vi "nii_read_data.vi"(8 "error in (no error)":errorcluster, 11 "file (use dialog)":path) -> (0 "error out":errorcluster, 2 "data value reference":refnum<data-value>, 3 "Data":T1 {"slice orientation" items=["transverse unflipped", "coronal unflipped", "sagittal unflipped", "transverse flipped", "coronal flipped", "sagittal flipped"]}, 4 "non-flip":bool, 5 "head":u8[](array[numeric]) format="%.0x")   [LabVIEW 2014]
uses:
  control/head_data.ctl
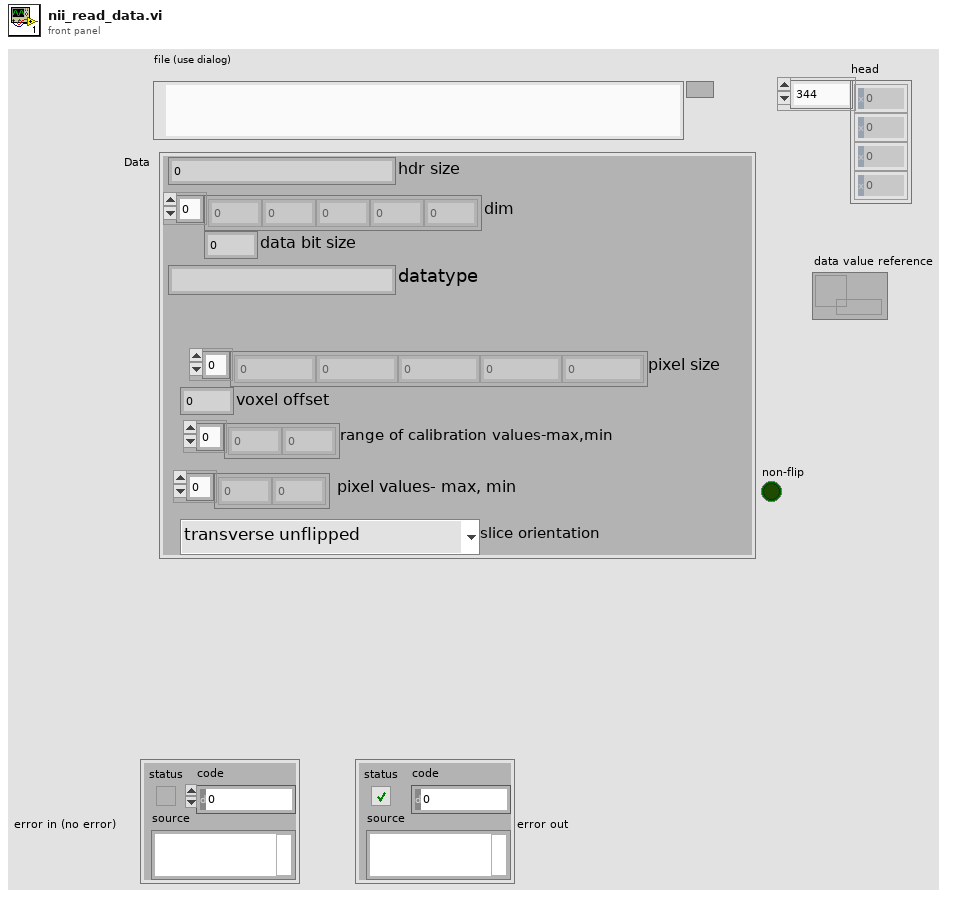
[diagram p1: front panel]
types:
  T1 = typedef "head_data.ctl" = cluster{"hdr size":i32, "dim":i32[], "data bit size":i32, "datatype":string, "pixel size ":sgl[], "voxel offset":sgl, "range of calibration values-max,min":sgl[], " pixel values- max, min":sgl[], "slice orientation":u16}
  T2 = enum16{"u_int8", "int8", "u_int16", "int16", "u_int32", "int32", "u_int64", "int64", "float", "double"}
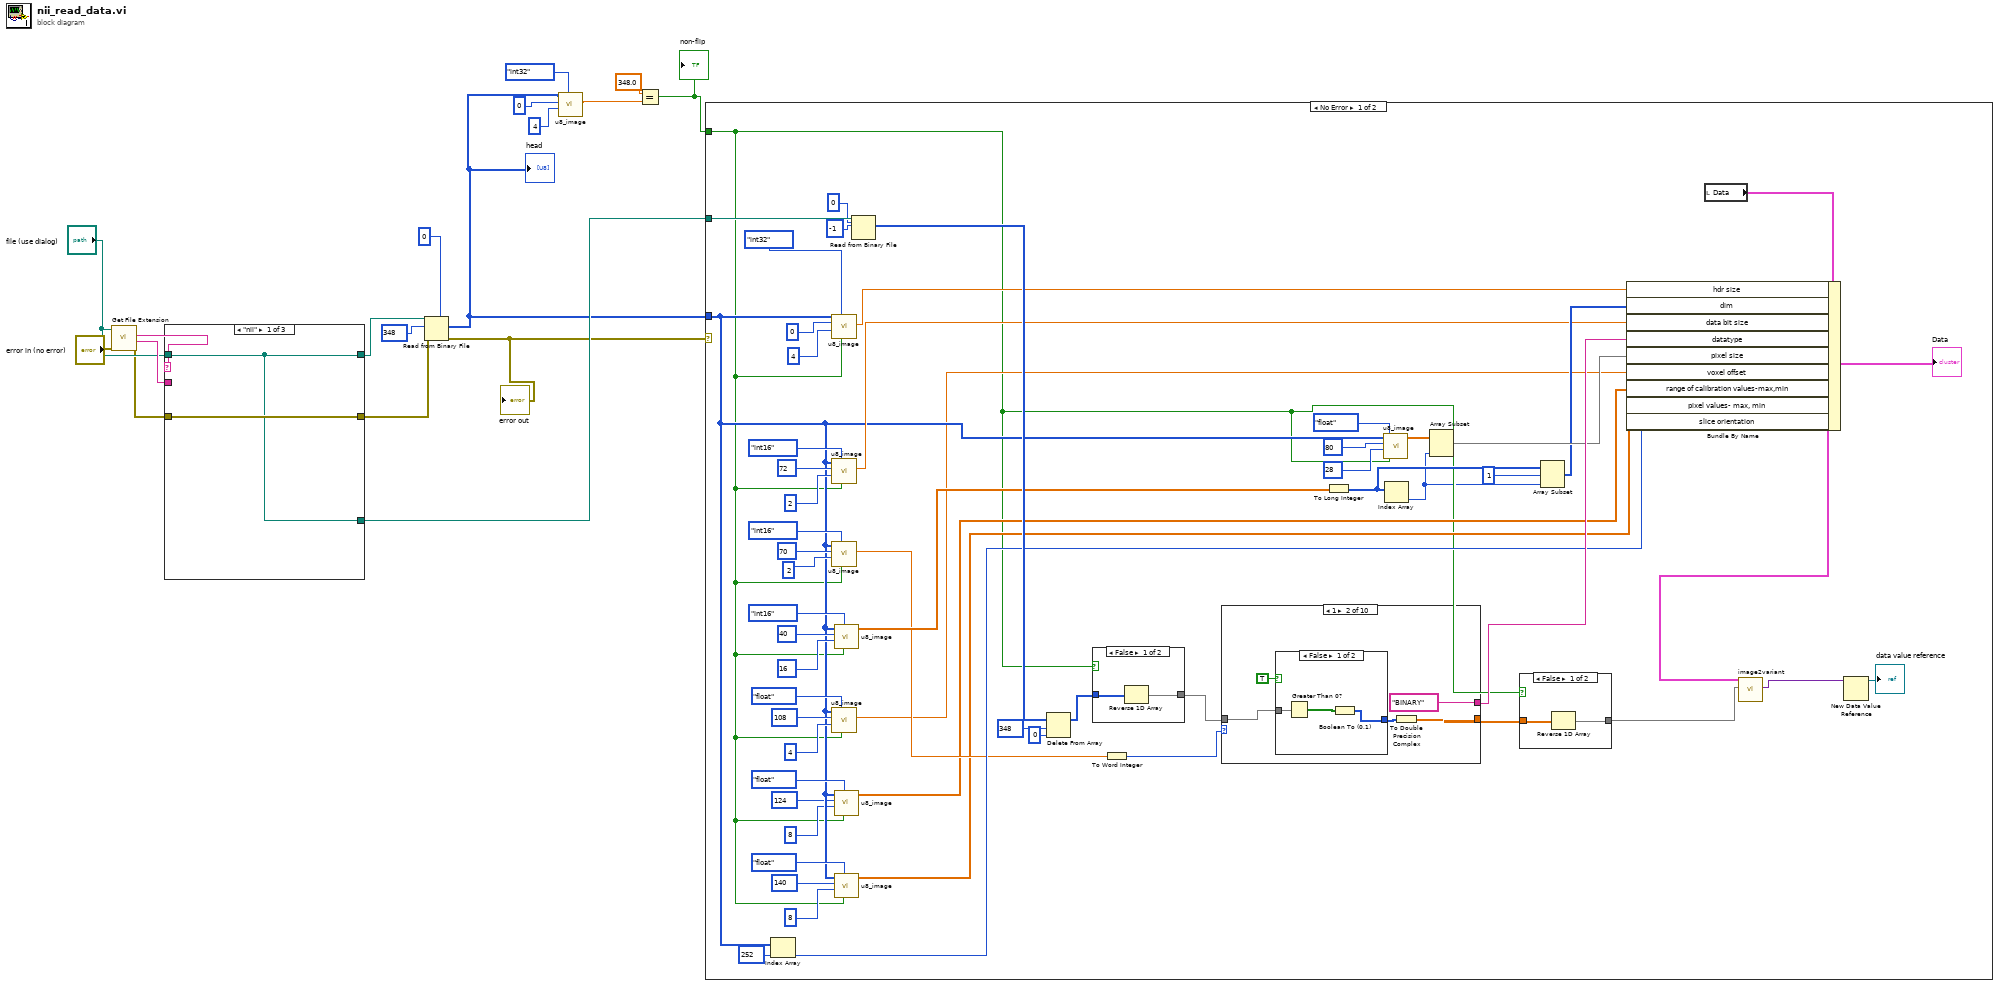
[diagram p0: block diagram]
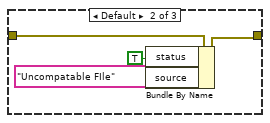
[diagram p2: hidden frame]
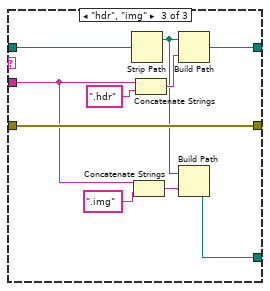
[diagram p3: hidden frame]
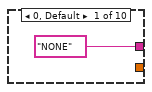
[diagram p6: hidden frame]
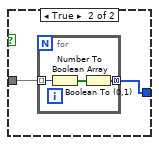
[diagram p7: hidden frame]
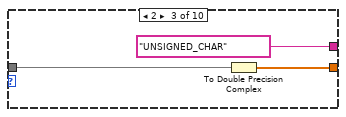
[diagram p8: hidden frame]
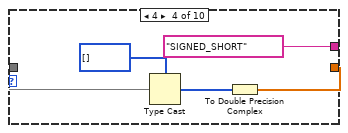
[diagram p9: hidden frame]
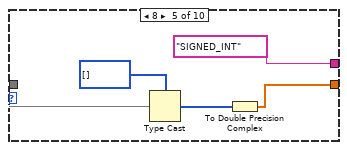
[diagram p10: hidden frame]
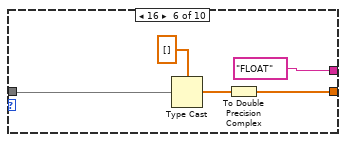
[diagram p11: hidden frame]
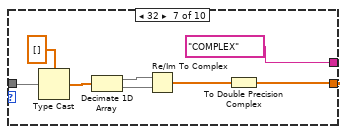
[diagram p12: hidden frame]
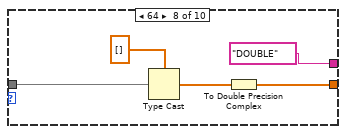
[diagram p13: hidden frame]
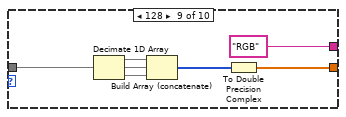
[diagram p14: hidden frame]
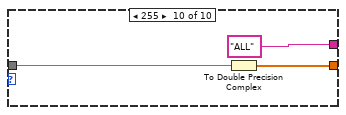
[diagram p15: hidden frame]
diagram:
  n1 = call <vilib>:"Get File Extension.vi"("error in (no error)"="error in (no error)", "file"="file (use dialog)") -> ("error out"=w14:errorcluster, "filename without extension"=w17:string, "lowercase file extension"=w18:string)  [unwired: 6 in, 1 out]
  n2 = case shown="\"nii\"" w18 {
    tunnel: "file (use dialog)" -> [w19 _ w30]
    tunnel: [w19 _ w32] -> w10
    tunnel: w17 -> [_ _ w26]
    tunnel: [w20 w23 w31] -> w15
    tunnel: w14 -> [w20 w24 w31]
    tunnel: [w19 _ w25] -> w12
    frame "nii" {
    }
    frame Default {
      n3 = Bundle By Name(cluster=w24, "status"=TRUE, "source"="Uncompatable FIle") -> (w23:errorcluster)
    }
    frame "hdr", "img" {
      n4 = Strip Path(path=w30) -> (stripped path=w29:path)  [unwired: 1 out]
      n5 = Concatenate Strings(w26, ".img" ("string")) -> (w28:string)
      n6 = Concatenate Strings(w26, ".hdr" ("string")) -> (w33:string)
      n7 = Build Path(base path=w29, name or relative path=w33) -> (appended path=w32:path)
      n8 = Build Path(base path=w29, name or relative path=w28) -> (appended path=w25:path)
    }
  }
  n9 = Read from Binary File(5:u8 0, 8:w15, 10:348 ("count (1)"), 11:w10) -> (0:w9:errorcluster, 2:w5:u8[])  [unwired: 2 in, 2 out]
  "error out" <- w9
  "head" <- w5
  n10 = call "u8_image.vi"("Enum"=T2."int32", "length"=4, "index"=0, "array"=w5) -> ("Numeric"=w3:dbl)  [unwired: 6 in, 1 out]
  n11 = Equal?(x=348.0, y=w3) -> (x = y?=w6:bool)
  "non-flip" <- w6
  n12 = case shown="No Error" w9 {
    tunnel: w5 -> [w49 _]
    tunnel: w12 -> [w91 _]
    tunnel: w6 -> [w41 _]
    frame No Error {
      n13 = Index Array(array=w49, index=252) -> (element=w83:u8)
      n14 = call "u8_image.vi"("non-flip"=w41, "Enum"=T2."int32", "length"=4, "index"=0, "array"=w49) -> ("Numeric"=w77:dbl)  [unwired: 5 in, 1 out]
      n15 = call "u8_image.vi"("non-flip"=w41, "Enum"=T2."int16", "length"=2, "index"=72, "array"=w49) -> ("Numeric"=w68:dbl)  [unwired: 5 in, 1 out]
      n16 = call "u8_image.vi"("non-flip"=w41, "Enum"=T2."int16", "length"=2, "index"=70, "array"=w49) -> ("Numeric"=w64:dbl)  [unwired: 5 in, 1 out]
      n17 = call "u8_image.vi"("non-flip"=w41, "Enum"=T2."float", "length"=4, "index"=108, "array"=w49) -> ("Numeric"=w46:dbl)  [unwired: 5 in, 1 out]
      n18 = call "u8_image.vi"("non-flip"=w41, "Enum"=T2."int16", "length"=16, "index"=40, "array"=w49) -> ("Array"=w74:dbl[])  [unwired: 5 in, 1 out]
      n19 = call "u8_image.vi"("non-flip"=w41, "Enum"=T2."float", "length"=8, "index"=124, "array"=w49) -> ("Array"=w50:dbl[])  [unwired: 5 in, 1 out]
      n20 = call "u8_image.vi"("non-flip"=w41, "Enum"=T2."float", "length"=8, "index"=140, "array"=w49) -> ("Array"=w53:dbl[])  [unwired: 5 in, 1 out]
      n21 = Read from Binary File(5:u8 0 ("default value 1"), 10:-1 ("count (1)"), 11:w91) -> (2:w88:u8[])  [unwired: 3 in, 3 out]
      n22 = Delete From Array(array=w88, length=348, index=0) -> (array with subset deleted=w44:u8[])  [unwired: 1 out]
      n23 = case shown="False" w41 {
        tunnel: [w95 w97] -> w43
        tunnel: w44 -> [w96 w97]
        frame False {
          n24 = Reverse 1D Array(array=w96) -> (reversed array=w95:u8[])
        }
        frame True {
        }
      }
      n25 = To Word Integer(number=w64) -> (16bit integer=w63:i16)
      n26 = case shown="1" w63 {
        tunnel: ["NONE" "BINARY" "UNSIGNED_CHAR" "SIGNED_SHORT" "SIGNED_INT" "FLOAT" "COMPLEX" "DOUBLE" "RGB" "ALL"] -> w87
        tunnel: [_ w102 w113 w118 w123 w128 w133 w141 w144 w150] -> w42
        tunnel: w43 -> [_ w101 w112 w117 w121 w125 w130 w138 w145 w151]
        frame 0, Default {
        }
        frame 1 {
          n27 = case shown="False" TRUE {
            tunnel: w101 -> [w105 w108]
            tunnel: [w104 w107] -> w100
            frame False {
              n28 = Greater Than 0?(x=w105) -> (x > 0?=w106:bool[])
              n29 = Boolean To (0,1)(Boolean=w106) -> (0, 1=w104:i16[])
            }
            frame True {
              n30 = for {
                tunnel: w108 -> [w111] mode=indexing
                tunnel: [w109] -> w107 mode=concatenating
                n31 = Number To Boolean Array(number=w111) -> (Boolean array=w110:bool[])
                n32 = Boolean To (0,1)(Boolean=w110) -> (0, 1=w109:i16[])
              }
            }
          }
          n33 = To Double Precision Complex(1:w100) -> (0:w102:cdb[])
        }
        frame 2 {
          n34 = To Double Precision Complex(1:w112) -> (0:w113:cdb[])
        }
        frame 4 {
          n35 = Type Cast(type=i16[] [], x=w117) -> (*(type *) &x=w116:i16[])
          n36 = To Double Precision Complex(1:w116) -> (0:w118:cdb[])
        }
        frame 8 {
          n37 = Type Cast(type=i32[] [], x=w121) -> (*(type *) &x=w120:i32[])
          n38 = To Double Precision Complex(1:w120) -> (0:w123:cdb[])
        }
        frame 16 {
          n39 = Type Cast(type=sgl[] [], x=w125) -> (*(type *) &x=w126:sgl[])
          n40 = To Double Precision Complex(1:w126) -> (0:w128:cdb[])
        }
        frame 32 {
          n41 = Type Cast(type=sgl[] [], x=w130) -> (*(type *) &x=w131:sgl[])
          n42 = Decimate 1D Array(w131) -> (w136:sgl[], w135:sgl[])
          n43 = Re/Im To Complex(1:w135, 2:w136) -> (0:w134:csg[])
          n44 = To Double Precision Complex(1:w134) -> (0:w133:cdb[])
        }
        frame 64 {
          n45 = Type Cast(type=dbl[] [], x=w138) -> (*(type *) &x=w139:dbl[])
          n46 = To Double Precision Complex(1:w139) -> (0:w141:cdb[])
        }
        frame 128 {
          n47 = Decimate 1D Array(w145) -> (w148:u8[], w147:u8[], w146:u8[])
          n48 = Build Array (concatenate)(w148, w147, w146) -> (w143:u8[])
          n49 = To Double Precision Complex(1:w143) -> (0:w144:cdb[])
        }
        frame 255 {
          n50 = To Double Precision Complex(1:w151) -> (0:w150:cdb[])
        }
      }
      n51 = To Long Integer(number=w74) -> (32bit integer=w80:i32[])
      n52 = call "u8_image.vi"("non-flip"=w41, "Enum"=T2."float", "length"=28, "index"=80, "array"=w49) -> ("Array"=w60:dbl[])  [unwired: 5 in, 1 out]
      n53 = Index Array(array=w80) -> (element=w40:i32)  [unwired: 1 in]
      n54 = Array Subset(array=w60, length=w40) -> (w86:dbl[])  [unwired: 1 in]
      n55 = case shown="False" w41 {
        tunnel: [w92 w94] -> w37
        tunnel: w42 -> [w93 w94]
        frame False {
          n56 = Reverse 1D Array(array=w93) -> (reversed array=w92:cdb[])
        }
        frame True {
        }
      }
      n57 = Array Subset(array=w80, index=1, length=w40) -> (w81:i32[])
      n58 = local read "Data"() -> (w85:T1)
      n59 = Bundle By Name(cluster=w85, "hdr size"=w77, "dim"=w81, "data bit size"=w68, "datatype"=w87, "pixel size"=w86, "voxel offset"=w46, "range of calibration values-max,min"=w50, "pixel values- max, min"=w53, "slice orientation"=w83) -> (w38:T1)
      "Data" <- w38
      n60 = call "image2variant.vi"("image_1d"=w37, "Data"=w38) -> ("variant"=w36:variant)  [unwired: 9 in]
      n61 = New Data Value Reference(data value=w36) -> (data value reference=→"data value reference":refnum<data-value>)  [unwired: 1 in, 1 out]
    }
    frame Error {
    }
  }
